vi "Generate Row Cells.vi"(0 "PDF Report":refnum<class "PDF Report Class.lvclass">, 2 "Number Colum":u16, 7 "Row Borders":T1={"Row"={"From #"=0, "to #"=-1}, "Cell [ ]"=[]}, 11 "error in (no error)":errorcluster) -> (4 "PDF Report duplicate":refnum<class "PDF Report Class.lvclass">, 8 "Row format with ref":T18, 15 "error out":errorcluster)   [LabVIEW 2019]
doc: "Version 2.0\nDeveloped by Jean-Marc Simard\nCopyright © 2012, Exaprom Inc.\nAll rights reserved.\nLicense: BSD\n\nWith iTextSharp 4.1.6 (http://itextsharp.sourceforge.net)\nunder Mozilla Public License Version 1.1\n(http://www.mozilla.org/MPL/MPL-1.1.html)"
uses:
  <userlib>/Exaprom PDF/LV Class/PDF Report Class/PDF Report Class.lvclass
  <userlib>/Exaprom PDF/Controls/Table Controls/Cell Cluster.ctl
  C:/Program Files/National Instruments/LabVIEW 2019/user.lib/Exaprom PDF/DLL/itextsharp.dll
  DLL/itextsharp.dll
  <userlib>/Exaprom PDF/Controls/Text Controls/Unicode/Type and run direction.ctl
  <userlib>/Exaprom PDF/Controls/Table Controls/Cell Alignment 20px.ctl
  <userlib>/Exaprom PDF/Controls/Table Controls/Text vertical arrangement.ctl
  <userlib>/Exaprom PDF/Controls/Font Controls/Font size.ctl
  <userlib>/Exaprom PDF/Controls/Table Controls/One Row Appearance.ctl
  <userlib>/Exaprom PDF/Controls/Table Controls/Row from to.ctl
  <userlib>/Exaprom PDF/Controls/Table Controls/Cell, Alignment, LS and Font - hide Vmerge.ctl
  <userlib>/Exaprom PDF/Controls/Table Controls/Cell Type, Alignment and LS.ctl
  <userlib>/Exaprom PDF/Controls/Text Controls/Line spacing.ctl
  <userlib>/Exaprom PDF/Controls/Table Controls/Cell Appearance.ctl
  <userlib>/Exaprom PDF/Controls/Table Controls/Cell Border 20 px.ctl
  <userlib>/Exaprom PDF/Controls/Table Controls/Merge Horizontal.ctl
  <userlib>/Exaprom PDF/Controls/Table Controls/Merge Vertical.ctl
  <userlib>/Exaprom PDF/Controls/Font Controls/Font complete cluster.ctl
  <userlib>/Exaprom PDF/Controls/Font Controls/Font color.ctl
  <userlib>/Exaprom PDF/Controls/Font Controls/Type and encoding.ctl
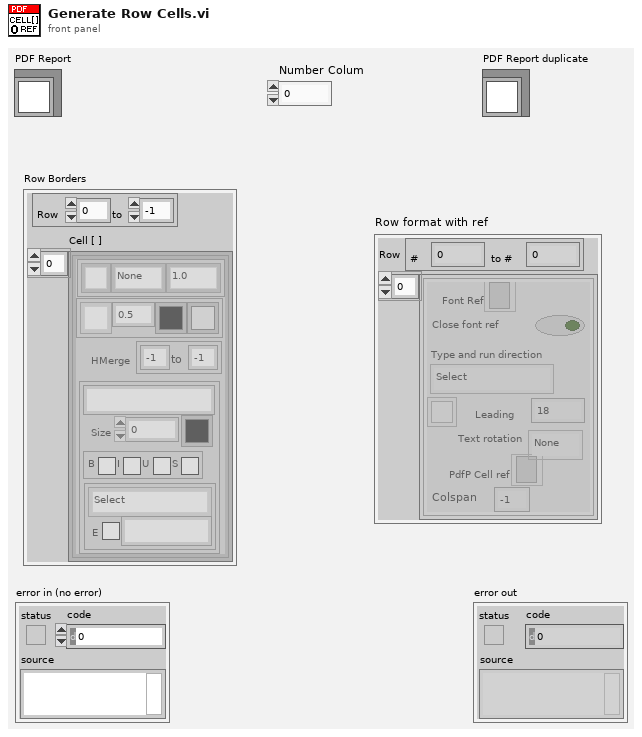
[diagram p1: front panel]
types:
  T1 = typedef "One Row Appearance.ctl" = cluster{"Row":T2, "Cell [ ]":T3[]}
  T2 = typedef "Row from to.ctl" = cluster{"From #":i16, "to #":i16}
  T3 = typedef "Cell, Alignment, LS and Font - hide Vmerge.ctl" = cluster{"Text":T4, "Cell Appearance":T8, "HMerge":T10, "VMerge":T11, "Font":T12}
  T4 = typedef "Cell Type, Alignment and LS.ctl" = cluster{"Cell Alignment":T5, "Text rotation":T6, "Line spacing":T7}
  T5 = typedef "Cell Alignment 20px.ctl" = u16
  T6 = typedef "Text vertical arrangement.ctl" = enum16{"None", "Clockwise", "Counterclockwise"}
  T7 = typedef "Line spacing.ctl" = enum16{"Select", "1.0", "1.5", "2.0"}
  T8 = typedef "Cell Appearance.ctl" = cluster{"Border":T9, "Thickness":sgl, "Color":u32, "BG":u32}
  T9 = typedef "Cell Border 20 px.ctl" = u16
  T10 = typedef "Merge Horizontal.ctl" = cluster{"From":i8, "to":i8}
  T11 = typedef "Merge Vertical.ctl" = cluster{"From":i8, "to":i8}
  T12 = typedef "Font complete cluster.ctl" = cluster{"Name":string, "Size":T13, "Color":T14, "Style":cluster{"Bold":bool, "Italic":bool, "Underline":bool, "Strikeout":bool}, "Type":T15}
  T13 = typedef "Font size.ctl" = sgl
  T14 = typedef "Font color.ctl" = u32
  T15 = typedef "Type and encoding.ctl" = cluster{"Type&direction":T16, "Embedded":bool, "Encoding":string}
  T16 = typedef "Type and run direction.ctl" = enum16{"Select", "ASCII", "UTF-16", "UTF-16 (default)", "UTF-16 (LTR)", "UTF-16 (RTL)"}
  T17 = typedef "Cell Cluster.ctl" = cluster{"Font Ref":refnum<k24>, "Close font ref":bool, "Type and run direction":T16, "Cell Alignment":T5, "Text rotation":T6, "Leading":T13, "PdfP Cell ref":refnum<k24>, "Colspan":i8}
  T18 = cluster{"Row":cluster{"#":i16, "to #":i16}, "Cell [ ]":T17[]}
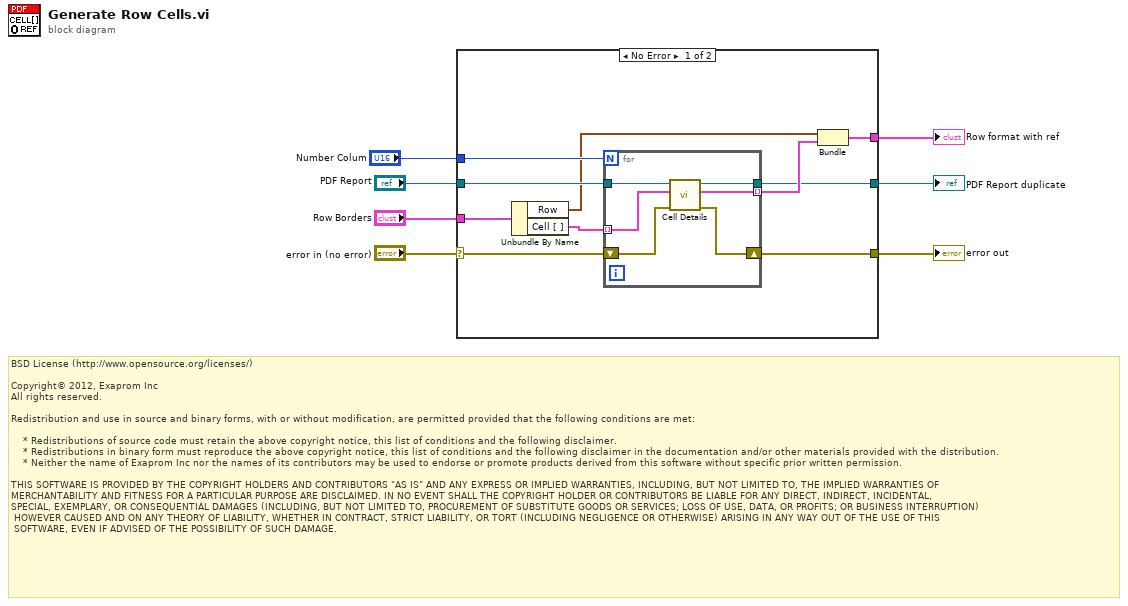
[diagram p0: block diagram]
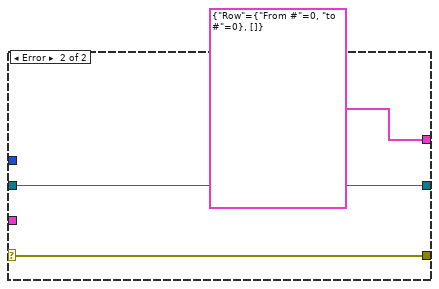
[diagram p2: hidden frame]
diagram:
  # "BSD License (http://www.opensource.org/licenses/)\n\nCopyright© 2012, Exaprom Inc\nAll rights reserved.\n\nRedistribution and use in source and binary forms, with or without modification, are permitted provided that the following conditions are met:\n\n    * Redistributions of source code must retain the above copyright notice, this list of conditions and the following disclaimer.\n    * Redistributions in binary form must reproduce the above copyright notice, this list of conditions and the following disclaimer in the documentation and/or other materials provided with the distribution.\n    * Neither the name of Exaprom Inc nor the names of its contributors may be used to endorse or promote products derived from this software without specific prior written permission.\n\nTHIS SOFTWARE IS PROVIDED BY THE COPYRIGHT HOLDERS AND CONTRIBUTORS \"AS IS\" AND ANY EXPRESS OR IMPLIED WARRANTIES, INCLUDING, BUT NOT LIMITED TO, THE IMPLIED WARRANTIES OF \nMERCHANTABILITY AND FITNESS FOR A PARTICULAR PURPOSE ARE DISCLAIMED. IN NO EVENT SHALL THE COPYRIGHT HOLDER OR CONTRIBUTORS BE LIABLE FOR ANY DIRECT, INDIRECT, INCIDENTAL,\nSPECIAL, EXEMPLARY, OR CONSEQUENTIAL DAMAGES (INCLUDING, BUT NOT LIMITED TO, PROCUREMENT OF SUBSTITUTE GOODS OR SERVICES; LOSS OF USE, DATA, OR PROFITS; OR BUSINESS INTERRUPTION)\n HOWEVER CAUSED AND ON ANY THEORY OF LIABILITY, WHETHER IN CONTRACT, STRICT LIABILITY, OR TORT (INCLUDING NEGLIGENCE OR OTHERWISE) ARISING IN ANY WAY OUT OF THE USE OF THIS\n SOFTWARE, EVEN IF ADVISED OF THE POSSIBILITY OF SUCH DAMAGE."
  n1 = case shown="No Error" "error in (no error)" {
    selector: "error in (no error)" -> [w14 w26]
    tunnel: "PDF Report" -> [w17 w24]
    tunnel: [w15 cluster{"Row":T2, T17[]} {"Row"={"From #"=0, "to #"=0}, []}] -> w7
    tunnel: [w13 w26] -> w5
    tunnel: "Number Colum" -> [w12 _]
    tunnel: "Row Borders" -> [w11 _]
    tunnel: [w8 w24] -> w1
    frame No Error {
      n2 = Unbundle By Name(w11) -> ("Row"=w9:T2, "Cell [ ]"=w10:T3[])
      n3 = for {
        N: w12 -> [_]
        tunnel: w17 -> [w23]
        tunnel: w10 -> [w21] mode=indexing
        shift-right: [w20] -> w13
        shift-left: w14 -> [w22]
        tunnel: [w19] -> w16 mode=indexing
        tunnel: [w18] -> w8
        n4 = call <userlib>:"Cell Details.vi"("error in (no error)"=w22, "Cell, Alignment, LS and Font"=w21, "PDF Report"=w23) -> ("error out"=w20:errorcluster, "Cell Cluster"=w19:T17, "PDF Report duplicate"=w18:refnum<class "PDF Report Class.lvclass">)  [unwired: 6 out]
      }
      n5 = Bundle("Row"=w9, w16) -> (w15:cluster{"Row":T2, T17[]})  [unwired: 1 out]
    }
    frame Error {
    }
  }
  "PDF Report duplicate" <- w1
  "error out" <- w5
  "Row format with ref" <- w7
